vi "Init.vi"(8 "error in (no error)":errorcluster, 10 "Address":string, 11 "Hamamatsu_Camera in":refnum<class "Hamamatsu_Camera.lvclass">) -> (0 "error out":errorcluster, 3 "Hamamatsu_Camera out":refnum<class "Hamamatsu_Camera.lvclass">)   [LabVIEW 2023, in "Hamamatsu_Camera.lvlib" / "Hamamatsu_Camera.lvclass"]
uses:
  Hamamatsu_Camera.lvclass
  typedefs/instrumentType.ctl
  typedefs/typedefs.lvlib
  <vilib>/ActorFramework/Actor/Actor.lvclass
  Interfaces/InitDeinitInterface/InitDeinitComm Messages/InitDone Msg/InitDone Msg.lvclass
  C:/Program Files/National Instruments/LabVIEW 2023/vi.lib/ActorFramework/Actor/Actor.lvclass
  C:/Users/quantum/Documents/LVDAQ/ConcreteClasses/ConcreteInstrumentClasses/CameraClasses/Hama_LV/HamaCam/Hamamatsu_Camera.lvclass
  C:/Users/quantum/Documents/LVDAQ/Interfaces/InitDeinitInterface/InitDeinit/InitDeinit.lvclass
  C:/Users/quantum/Documents/LVDAQ/Interfaces/AbstractInstrumentClasses/Cameras_LV/CameraInterface/CameraInterface.lvclass
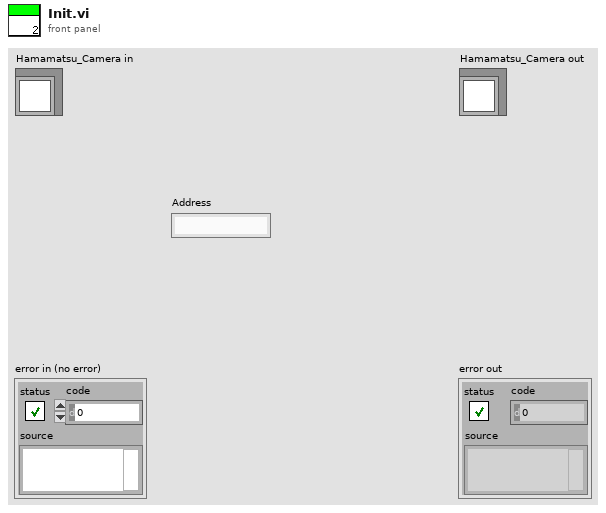
[diagram p1: front panel]
types:
  T1 = typedef "typedefs.lvlib/instrumentType.ctl" = enum16{"Spectrometer", "Camera", "Stepper", "Piezo"}
  T2 = cluster{"address type":enum16{"VISA", "Index"}, "Address":string, "instrument type":T1}
  T3 = typedef "typedefs.lvlib/Camera_Init_Params.ctl" = cluster{"Exposure":dbl, "Gain":dbl, "Image XDim":u16, "Image YDim":u16, "Pixel Size":sgl}
  T4 = cluster{"Instr Error":errorcluster, "CameraData":T3, "Address":cluster{"address type":enum16{"VISA", "Index"}, "Address":string, "instrument type":T1}}
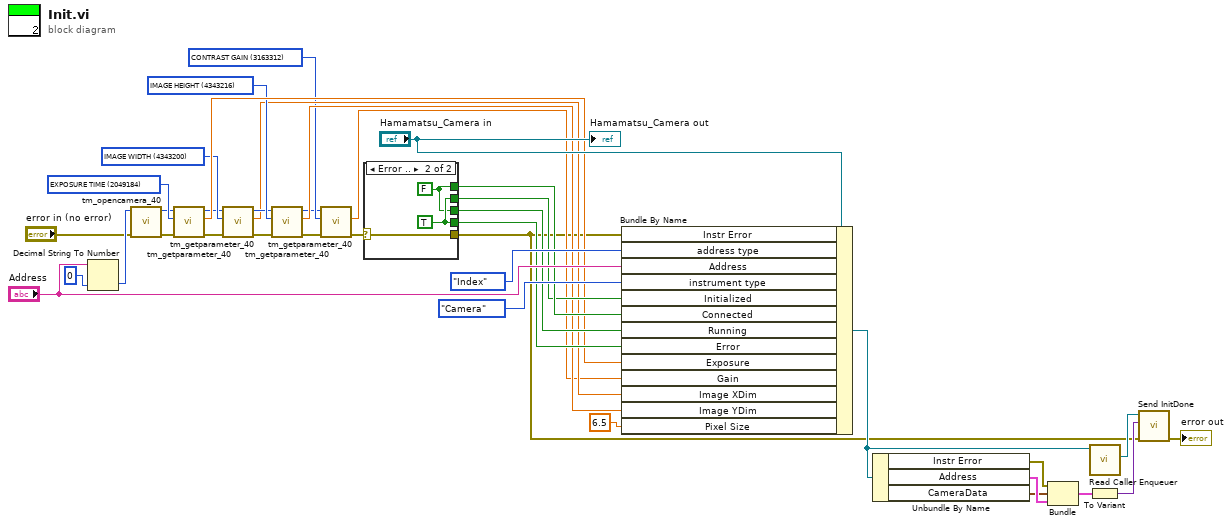
[diagram p0: block diagram]
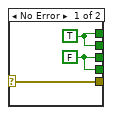
[diagram p2: hidden frame]
diagram:
  w17 = u32 3163312 items=["SENSOR MODE"=4212128, "SENSOR MODE LINE BUNDLE HEIGHT"=4212192, "READOUT DIRECTION"=4211904, "BIT PER CHANNEL"=4342976, "EXPOSURE TIME"=2049184, "CONTRAST GAIN"=3163312, "BINNING"=4215968, "TIMING READOUT TIME"=4223904, "INTERNAL FRAME RATE"=4225952, "INTERNAL FRAME INTERVAL"=4225968, "INTERNAL LINE SPEED"=4226000, "IMAGE WIDTH"=4343200, "IMAGE HEIGHT"=4343216, "IMAGE ROWBYTES"=4343232, "IMAGE FRAMEBYTES"=4343248, "IMAGE PIXEL TYPE"=4343296] ("Parameter")
  w22 = u32 4343216 items=["SENSOR MODE"=4212128, "SENSOR MODE LINE BUNDLE HEIGHT"=4212192, "READOUT DIRECTION"=4211904, "BIT PER CHANNEL"=4342976, "EXPOSURE TIME"=2049184, "CONTRAST GAIN"=3163312, "BINNING"=4215968, "TIMING READOUT TIME"=4223904, "INTERNAL FRAME RATE"=4225952, "INTERNAL FRAME INTERVAL"=4225968, "INTERNAL LINE SPEED"=4226000, "IMAGE WIDTH"=4343200, "IMAGE HEIGHT"=4343216, "IMAGE ROWBYTES"=4343232, "IMAGE FRAMEBYTES"=4343248, "IMAGE PIXEL TYPE"=4343296] ("Parameter")
  w23 = u32 4343200 items=["SENSOR MODE"=4212128, "SENSOR MODE LINE BUNDLE HEIGHT"=4212192, "READOUT DIRECTION"=4211904, "BIT PER CHANNEL"=4342976, "EXPOSURE TIME"=2049184, "CONTRAST GAIN"=3163312, "BINNING"=4215968, "TIMING READOUT TIME"=4223904, "INTERNAL FRAME RATE"=4225952, "INTERNAL FRAME INTERVAL"=4225968, "INTERNAL LINE SPEED"=4226000, "IMAGE WIDTH"=4343200, "IMAGE HEIGHT"=4343216, "IMAGE ROWBYTES"=4343232, "IMAGE FRAMEBYTES"=4343248, "IMAGE PIXEL TYPE"=4343296] ("Parameter")
  w27 = u32 2049184 items=["SENSOR MODE"=4212128, "SENSOR MODE LINE BUNDLE HEIGHT"=4212192, "READOUT DIRECTION"=4211904, "BIT PER CHANNEL"=4342976, "EXPOSURE TIME"=2049184, "CONTRAST GAIN"=3163312, "BINNING"=4215968, "TIMING READOUT TIME"=4223904, "INTERNAL FRAME RATE"=4225952, "INTERNAL FRAME INTERVAL"=4225968, "INTERNAL LINE SPEED"=4226000, "IMAGE WIDTH"=4343200, "IMAGE HEIGHT"=4343216, "IMAGE ROWBYTES"=4343232, "IMAGE FRAMEBYTES"=4343248, "IMAGE PIXEL TYPE"=4343296] ("Parameter")
  n1 = Decimal String To Number(string="Address", default (0L)=u32 0 ("default (0 I32)")) -> (number=w38:u32)  [unwired: 1 in, 1 out]
  n2 = call "tm_opencamera_40.vi"("error in (no error)"="error in (no error)", "Camera Index"=w38) -> ("error out"=w24:errorcluster, "Handle out"=w26:u32)  [unwired: 7 in, 1 out]
  n3 = call "tm_getparameter_40.vi"("error in (no error)"=w24, "Parameter"=w27, "Handle in"=w26) -> ("error out"=w13:errorcluster, "Value out"=w25:dbl, "Handle out"=w20:u32)  [unwired: 6 in]
  n4 = call "tm_getparameter_40.vi"("error in (no error)"=w13, "Parameter"=w23, "Handle in"=w20) -> ("error out"=w15:errorcluster, "Value out"=w18:dbl, "Handle out"=w21:u32)  [unwired: 6 in]
  n5 = call "tm_getparameter_40.vi"("error in (no error)"=w15, "Parameter"=w22, "Handle in"=w21) -> ("error out"=w14:errorcluster, "Value out"=w19:dbl, "Handle out"=w11:u32)  [unwired: 6 in]
  n6 = call "tm_getparameter_40.vi"("error in (no error)"=w14, "Parameter"=w17, "Handle in"=w11) -> ("error out"=w12:errorcluster, "Value out"=w16:dbl)  [unwired: 6 in, 1 out]
  n7 = case shown="Error .." w12 {
    selector: w12 -> [w41 w42]
    tunnel: [w41 w42] -> w2
    tunnel: [w39 w43] -> w31
    tunnel: [w39 w44] -> w30
    tunnel: [w40 w43] -> w29
    tunnel: [w40 w44] -> w28
    frame No Error {
      w40 = FALSE ("InstrumentData.CurrentState.Connected")
      w39 = TRUE ("InstrumentData.CurrentState.Connected")
    }
    frame Error {
      w43 = FALSE ("InstrumentData.CurrentState.Connected")
      w44 = TRUE ("InstrumentData.CurrentState.Connected")
    }
  }
  n8 = Bundle By Name(cluster="Hamamatsu_Camera in", "Instr Error"=w2, "address type"=enum16{"VISA", "Index"}."Index" ("InstrumentData.Address.address type"), "Address"="Address", "instrument type"=instrumentType."Camera" ("InstrumentData.Address.instrument type"), "Initialized"=w30, "Connected"=w31, "Running"=w29, "Error"=w28, "Exposure"=w25, "Gain"=w16, "Image XDim"=w18, "Image YDim"=w19, "Pixel Size"=sgl 6.5 ("CameraData.Pixel Size")) -> (w3:refnum<class "Hamamatsu_Camera.lvclass">)
  n9 = Unbundle By Name(w3) -> ("Instr Error"=w6:errorcluster, "Address"=w5:T2, "CameraData"=w4:T3)
  n10 = Bundle("Instr Error"=w6, "CameraData"=w4, "Address"=w5) -> (w7:T4)  [unwired: 1 in]
  n11 = call <vilib>:"Read Caller Enqueuer.vi"("Actor"=w3) -> ("Caller Enqueuer"=w9:refnum<class "Message Enqueuer.lvclass">)  [unwired: 10 in]
  n12 = To Variant(anything=w7) -> (Variant=w8:variant)
  n13 = call "Send InitDone.vi"("error in (no error)"=w2, "Variant"=w8, "Message Enqueuer"=w9) -> ("error out"=→"error out":errorcluster)  [unwired: 7 in, 1 out]
  "Hamamatsu_Camera out" <- "Hamamatsu_Camera in"
